vi "MSEncoder SubVI WfmCodeGen_ShowGraph.vi"(4 "progress refnum":refnum<vi>, 6 "system graph refnum":refnum<vi>, 7 "Graph Display":refnum<vi>, 8 "error in (no error)":errorcluster, 9 "X Scale.Range:Minimun":dbl format="%#_13g", 10 "X Scale.Range:Maximum":ext, 11 "Display queue in":refnum<queue>) -> (0 "error out":errorcluster)   [LabVIEW 2018, in "MSEncoder.lvclass"]
uses:
  MSEncoder.lvclass
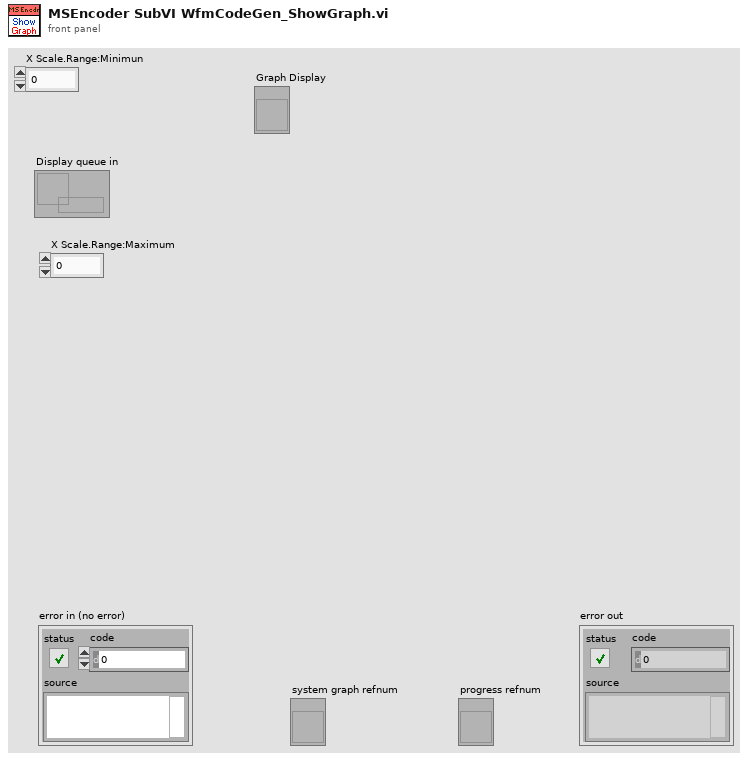
[diagram p1: front panel]
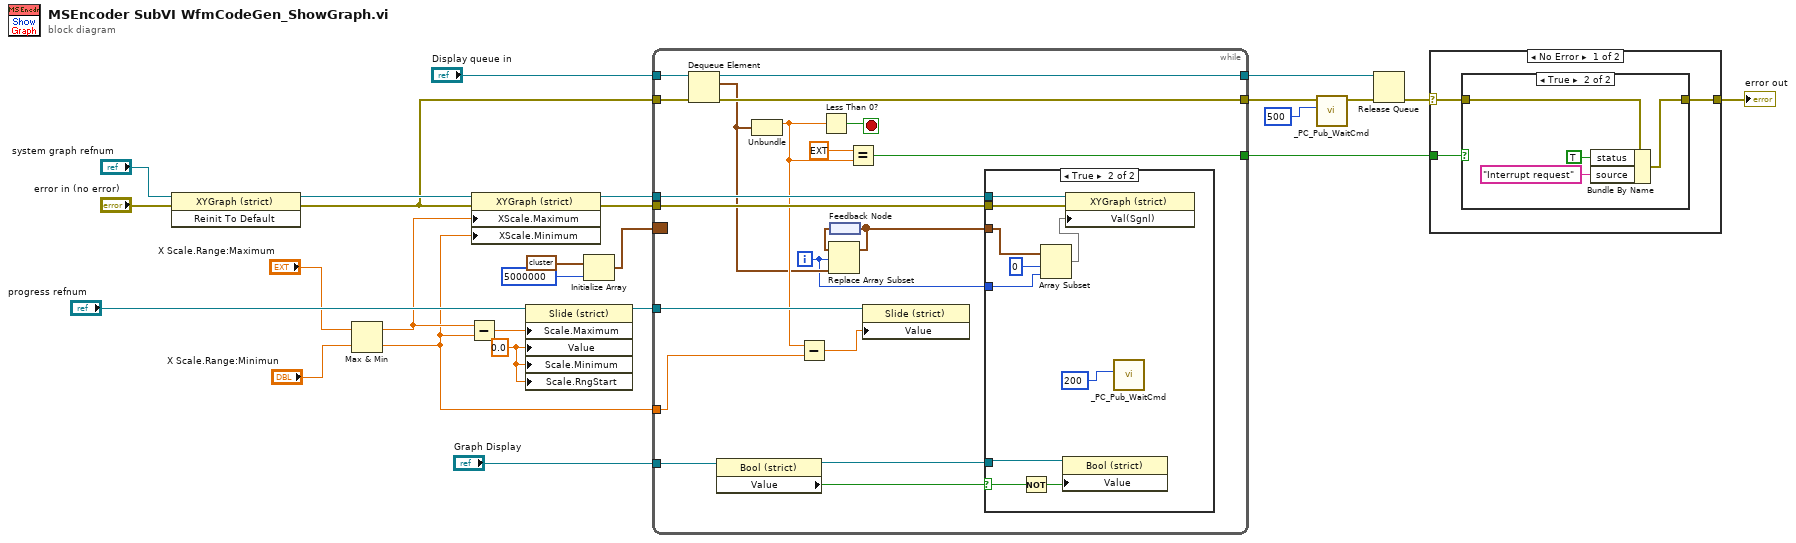
[diagram p0: block diagram]
diagram:
  w7 = 0.0 ("Value")
  n1 = invoke class="XYGraph (strict)" method="Reinit To Default"(reference="system graph refnum", error in="error in (no error)") -> (reference out=w18:refnum<vi>, error out=w16:errorcluster)  [unwired: 1 in, 1 out]
  n2 = Max & Min(x="X Scale.Range:Maximum", y="X Scale.Range:Minimun") -> (max(x,y)=w9:ext, min(x,y)=w6:ext)
  n3 = Subtract(x=w9, y=w6) -> (x-y=w8:ext)
  n4 = property class="XYGraph (strict)"(reference=w18, error in=w16, "XScale.Maximum"=w9, "XScale.Minimum"=w6) -> (reference out=w24:refnum<vi>, error out=w23:errorcluster)
  n5 = property class="Slide (strict)"(reference="progress refnum", "Scale.Maximum"=w8, "Value"=w7, "Scale.Minimum"=w7, "Scale.RngStart"=w7) -> (reference out=w25:refnum<vi>)  [unwired: 1 in, 1 out]
  n6 = Initialize Array(cluster{ext, ext} {0.0, 0.0}, 5000000 ("dimension size")) -> (w2:cluster{ext, ext}[])
  n7 = while {
    tunnel: "Display queue in" -> [w46]
    tunnel: w16 -> [w45]
    tunnel: [w44] -> w26
    tunnel: w25 -> [w43]
    tunnel: w24 -> [w42]
    tunnel: [w41] -> w22
    tunnel: w23 -> [w40]
    tunnel: [w35] -> w13
    tunnel: w6 -> [w39]
    tunnel: "Graph Display" -> [w34]
    border: w2 -> [_]
    i -> [w29]
    stop <- w36 stop-if-true
    n8 = Dequeue Element(queue=w46, error in (no error)=w45) -> (queue out=w44:refnum<queue>, element=w32:cluster{ext, "Amp2":ext}, error out=w41:errorcluster)  [unwired: 1 in, 1 out]
    n9 = property class="Bool (strict)"(reference=w34) -> (reference out=w27:refnum<vi>, "Value"=w28:bool)  [unwired: 1 in, 1 out]
    n10 = Unbundle(w32) -> (w37:ext)  [unwired: 1 out]
    n11 = Subtract(x=w37, y=w39) -> (x-y=w30:ext)
    n12 = Less Than 0?(x=w37) -> (x < 0?=w36:bool)
    n13 = feedback #1() -> (w33:cluster{ext, ext}[])
    n14 = Replace Array Subset(array=w33, new element=w32, index=w29) -> (w31:cluster{ext, ext}[])
    n15 = feedback-in #1(w31) -> ()
    n16 = Equal?(x=ext -1.0, y=w37) -> (x = y?=w35:bool)
    n17 = property class="Slide (strict)"(reference=w43, "Value"=w30) -> ()  [unwired: 1 in, 2 out]
    n18 = case shown="True" w28 {
      selector: w28 -> [_ w49]
      tunnel: w42 -> [_ w56]
      tunnel: w40 -> [_ w55]
      tunnel: w31 -> [_ w54]
      tunnel: w29 -> [_ w52]
      tunnel: w27 -> [_ w50]
      frame False {
      }
      frame True {
        n19 = Not(x=w49) -> (.not. x?=w48:bool)
        n20 = Array Subset(array=w54, index=0, length=w52) -> (w51:cluster{ext, ext}[])
        n21 = property class="Bool (strict)"(reference=w50, "Value"=w48) -> ()  [unwired: 1 in, 2 out]
        n22 = property class="XYGraph (strict)"(reference=w56, error in=w55, "Val(Sgnl)"=w51) -> ()  [unwired: 2 out]
        n23 = call "_PC_Pub_WaitCmd.vi"("milliseconds to wait"=u32 200) -> ()  [unwired: 10 in, 1 out]
      }
    }
  }
  n24 = call "_PC_Pub_WaitCmd.vi"("milliseconds to wait"=u32 500, "error in (no error)"=w22) -> ("error out"=w20:errorcluster)  [unwired: 9 in]
  n25 = Release Queue(queue=w26, error in (no error)=w20) -> (error out=w15:errorcluster)  [unwired: 1 in, 2 out]
  n26 = case shown="No Error" w15 {
    selector: w15 -> [w57 w65]
    tunnel: [w58 w65] -> w14
    tunnel: w13 -> [w59 _]
    frame No Error {
      n27 = case shown="True" w59 {
        tunnel: [w60 w61] -> w58
        tunnel: w57 -> [w60 w62]
        frame False {
        }
        frame True {
          n28 = Bundle By Name(cluster=w62, "status"=TRUE, "source"="Interrupt request") -> (w61:errorcluster)
        }
      }
    }
    frame Error {
    }
  }
  "error out" <- w14
